vi "GUI_Bella_Control_Center_OFI.vi"() -> ()   [LabVIEW 2020]
uses:
  Shared/GUI_Template/GUI_master/tcp_new_data_event.ctl
  Shared/GUI_Template/GUI_master/tcp new data cluster.ctl
  GUI_TestStand/Fire button.ctl
  Device Drivers/DG645/subVIs/TriggerSource_TypDef.ctl
  <vilib>/Utility/config.llb/Write Key (I32).vi
  <vilib>/Platform/browser.llb/Open URL in Default Browser (string).vi
  <vilib>/Utility/config.llb/NI_LVConfig.lvlib
panel:
  in  "value5::42":dbl=0.006 caption="1BL-2BL-\nSplitter-Rpcnt" min=-9999999.0 max=9999999.0 format="%#_6p"
  in  "value6::43":bool=TRUE caption="GhostFoil-In"
  in  "value5::43":bool=TRUE caption="1BL-Energy\nMeter-In"
  in  "value4::43":bool=TRUE caption="2BLFoil-In"
  in  "value3::43":bool=TRUE caption="1BLFoil-In"
  in  "value2::43":bool=TRUE caption="ClunkerIn"
  out "CurrentStatus":string
  in  "MoveStage":bool
  in  "Position.Ch1::44":dbl caption="Current Position" min=0.0 max=150.0
  in  "GUIdevice 44":string="STAGE-LT-Megattenuator"
  in  "GUIdevice 43":string="MANPAR-BELLA-OFI-Boolean"
  in  "GUIdevice 42":string="MANPAR-BELLA-OFI"
  in  "Pressure.device 2::39":dbl caption="Dopant pressure\nLow1down" min=-20.0 max=500.0 format="%.3f"
  out "HPD2 to match HPD":dbl
  in  "Save screenshots":bool
  out "error out":errorcluster
  out "Hpd pos for jet exit":dbl
  in  "value2::42":dbl=276.0 caption="jet exit on hpd for hexX=0" min=-9999999.0 max=9999999.0
  in  "GUIdevice 41":string="STAGE-PL1-JetLength"
  in  "position::41":dbl caption="Jet Length pos" min=0.0 max=50.0 format="%.1f"
  out "lp mode HPDplane\n - HPD ref pos":dbl
  out "height above jet":dbl
  in  "value3::42":dbl=2.6 caption="zpos for 0 above jet" min=-9999999.0 max=9999999.0
  out "HPD - focus":dbl
  in  "value1::42":dbl=230.0 caption="focus on HPD" min=-9999999.0 max=9999999.0
  out "1BL delay (ns)\n+ is 1BL after 2BL":dbl
  in  "Position.Axis 1::8":dbl caption="1BL delay (mm)" min=-500.0 max=500.0 format="%.1f"
  in  "GUIdevice 8":string="STAGE-LT-1BLDelay"
  in  "value4::42":dbl=0.006 caption="JetOnTime" min=-9999999.0 max=9999999.0 format="%#_6p"
  in  "Position.Channel 5::25":dbl caption="SMFiber (45in, 1out)" min=-60.0 max=55.0 format="%.1f"
  in  "value1::43":bool=TRUE caption="GasJetOn"
  in  "value0::43":bool=TRUE caption="ShotControl"
  in  "Thales.DIAG_CU_Output_Percent_1::37":dbl caption="Amp2 att (%)" min=1.0 max=100.0 step=500.0 format="%.2f"
  in  "GUIdevice 37":string="SVE-LT-Thales"
  in  "Pressure.device 1::39":dbl caption="Hydrogen pressure\nHigh500" min=-20.0 max=500.0 format="%.3f"
  in  "GUIdevice 39":string="PRC-PL1-HighPressure"
  in  "Scan":T1(ring)
  in  "LogTable":bool
  in  "New Google\nExpLog for new day?":bool=TRUE
  out "standard output":string
  in  "Create Log":bool caption="LogTable"
  in  "GUIdevice 38":string="STAGE-2BL-Compressor"
  in  "Position.Axis 1::38":dbl caption="Comp2 Translation" min=0.0 max=20.0 format="%.3f"
  in  "Position.Channel 5::31":T2(ring) caption="FROG foil"
  in  "Position.Channel 2::31":T2(ring) caption="Little Rick"
  in  "AnalogOutput.Channel 1::36":dbl caption="M4A att (V)" min=0.0 max=5.0 step=500.0 format="%.2f"
  in  "GUIdevice 36":string="ATT-2BL-M4A"
  in  "GUIdevice 35":string="ATT-2BL-DM"
  in  "AnalogOutput.Channel 1::35":dbl caption="2BL DM att (V)" min=0.0 max=5.0 step=500.0 format="%.2f"
  in  "Step size 2":dbl=20.0 caption="Step size" min=-22.0 max=22.0
  in  "Position.Axis 4::33":dbl caption="Holy M V F4" min=-100000.0 max=100000.0 step=500.0
  in  "Position.Axis 3::33":dbl caption="Holy M H F3" min=-1000000.0 max=1000000.0 step=500.0
  in  "Position.Axis 2::33":dbl caption="Bessel M3 V F2" min=-100000.0 max=100000.0 step=500.0
  in  "Position.Axis 1::33":dbl caption="Bessel M3 H F1" min=-100000.0 max=100000.0 step=500.0
  in  "GUIdevice 33":string="MCD-PL1-picosOFI1"
  in  "Delay.Ch B::32":dbl caption="jet open time B" min=-0.1 max=0.1 format="%.3p"
  in  "Delay.Ch A::32":dbl caption="jet open A" min=-0.1 max=0.1 format="%.3p"
  in  "GUIdevice 32":string="DDG-AA-SRSGasJet-645"
  in  "position::6":dbl caption="LPmode stage long (605 safe)" min=0.0 max=605.0 format="%.1f"
  in  "GUIdevice 6":string="STAGE-PL1-LPmodeLong"
  in  "EnableMotor::6":bool caption="LPmode motor \nstatus"
  in  "GUIdevice 4":string="STAGE-PL1-Capstage1"
  in  "GUIdevice 31":string="1WIRE-BELLA-Flipper"
  in  "Amplitude.Ch GH::10":dbl=-1.631e-06 caption="Shot Shutter V" min=0.5 max=5.0 format="%.1f"
  in  "Rate (Hz)":dbl=0.3
  out "Crystal2":enum16{"In", "Out", "Unknown"}(ring)
  in  "wangle::28":dbl caption="w" min=-2.0 max=2.0 step=0.01 format="%.5f"
  in  "vangle::28":dbl caption="v" min=-5.0 max=5.0 step=0.01 format="%.5f"
  in  "uangle::28":dbl caption="u" min=-1.0 max=1.0 step=0.01 format="%.5f"
  in  "ypos::28":dbl caption="y" min=-3.0 max=3.0 step=0.01 format="%.5f"
  in  "zpos::28":dbl caption="z" min=-12.5 max=12.5 step=0.01 format="%.5f"
  in  "xpos::28":dbl caption="x" min=-0.5 max=0.5 step=0.01 format="%.5f"
  in  "GUIdevice 28":string="HEX-PL1-2"
  in  "Position.Channel 1::25":dbl caption="LPmode kicker (~1in, 75out)" min=-75.0 max=79.0 format="%.1f"
  in  "GUIdevice 25":string="STAGE-PL1-Smaract"
  in  "Heater Alignment Directions":bool
  in  "Position.Axis 3::15":dbl caption="XY" min=-3.0 max=16.0 format="%.4f"
  in  "Position.Axis 2::15":dbl caption="Y" min=-3.0 max=17.0 format="%.4f"
  in  "Position.Axis 1::15":dbl caption="X" min=-3.0 max=13.0 format="%.4f"
  in  "GUIdevice 24":string="STAGE-HEAT-TL1"
  in  "Encoder position::23":dbl caption="position HPD2" min=0.0 max=600.0 format="%.1f"
  in  "position::3":dbl caption="position HPD" min=0.0 max=600.0 format="%.1f"
  in  "GUIdevice 23":string="STAGE-HPD-Far"
  in  "GUIdevice 22":string="MANPAR-BELLA-FireCont"
  in  "Allow Fire Continues":bool
  out "Fire continues Indicator":bool caption="firing"
  in  "Fire Button":T3=TRUE
  in  "Trigger.Source::10":T4 caption="SRS Trigger Mode"
  out "Absolute discharge timing":dbl caption="delay from pk" format="%#.3p"
  in  "Delay.Ch E::17":dbl caption="Timing box" min=-0.1 max=0.1 format="%.3p"
  in  "value0::22":bool caption="Fire continuosly"
  in  "GUIdevice 15":string="MCD-HEAT-ESP1"
  in  "GUIdevice 17":string="DDG-AA-SRS0"
  out "error IO 2":errorcluster
  out "fire::10":string
  out "tcp data event":T5
  in  "UDP error message":string
  in  "GUIdevice 13":string="DDG-AA-SRS2"
  in  "GUIdevice 2":string="MANPAR-BELLA-General"
  in  "GUIdevice 10":string="DDG-AA-ShotCntrl"
  in  "GUIdevice 1":string="HEX-PL1-1"
  in  "GUIdevice 3":string="STAGE-HPD-Tel"
  in  "<command>::1":bool caption="ABORT\nHEXAPOD"
  in  "Step size":dbl min=-22.0 max=22.0 format="%.5f"
  in  "wangle::1":dbl caption="w (F11 F12)" min=-6.0 max=6.0 step=0.01 format="%.5f"
  in  "vangle::1":dbl caption="v (F9 F10)" min=-6.0 max=6.0 step=0.01 format="%.5f"
  in  "uangle::1":dbl caption="u (F7 F8)" min=-6.0 max=6.0 step=0.01 format="%.5f"
  in  "ypos::1":dbl caption="y (F3 F4)" min=-8.0 max=8.0 step=0.01 format="%.5f"
  in  "zpos::1":dbl caption="z (PgU PgD)" min=-12.0 max=15.0 step=0.01 format="%.5f"
  in  "xpos::1":dbl caption="x (F1 F2)" min=-25.0 max=22.0 step=0.01 format="%.5f"
  in  "Position.Axis 1::9":dbl caption="Comp1 Translation" min=-50.0 max=50.0 format="%.3f"
  in  "GUIdevice 9":string="STAGE-1BL-Compression"
  in  "stop":bool
  # "BELLA CONTROL CENTER"
  # "HEX 1 JET"
  # "HEX 2 Axicon"
  # "PICOS"
  # "DG"
  # "Jet"
  # "Discharge timing (s)"
  # "1wire"
  # "Heater timing (s)"
  # "\"-x\" is laser propagation direction"
  # "Scan"
  # "HPD Stage"
  # "PL1 stages"
  # "Megattenuator Stage"
  # "needs manpar-bella-ofi on\nMANPAR-BELLA-OFI-Boolean"
  # "Attenuate"
  # "OUT"
  # "IN"
  # "Compressors"
  # "Heater Alignment"
  # "Heat ESP0"
  # "Heat ESP1"
  # "Heat Pico"
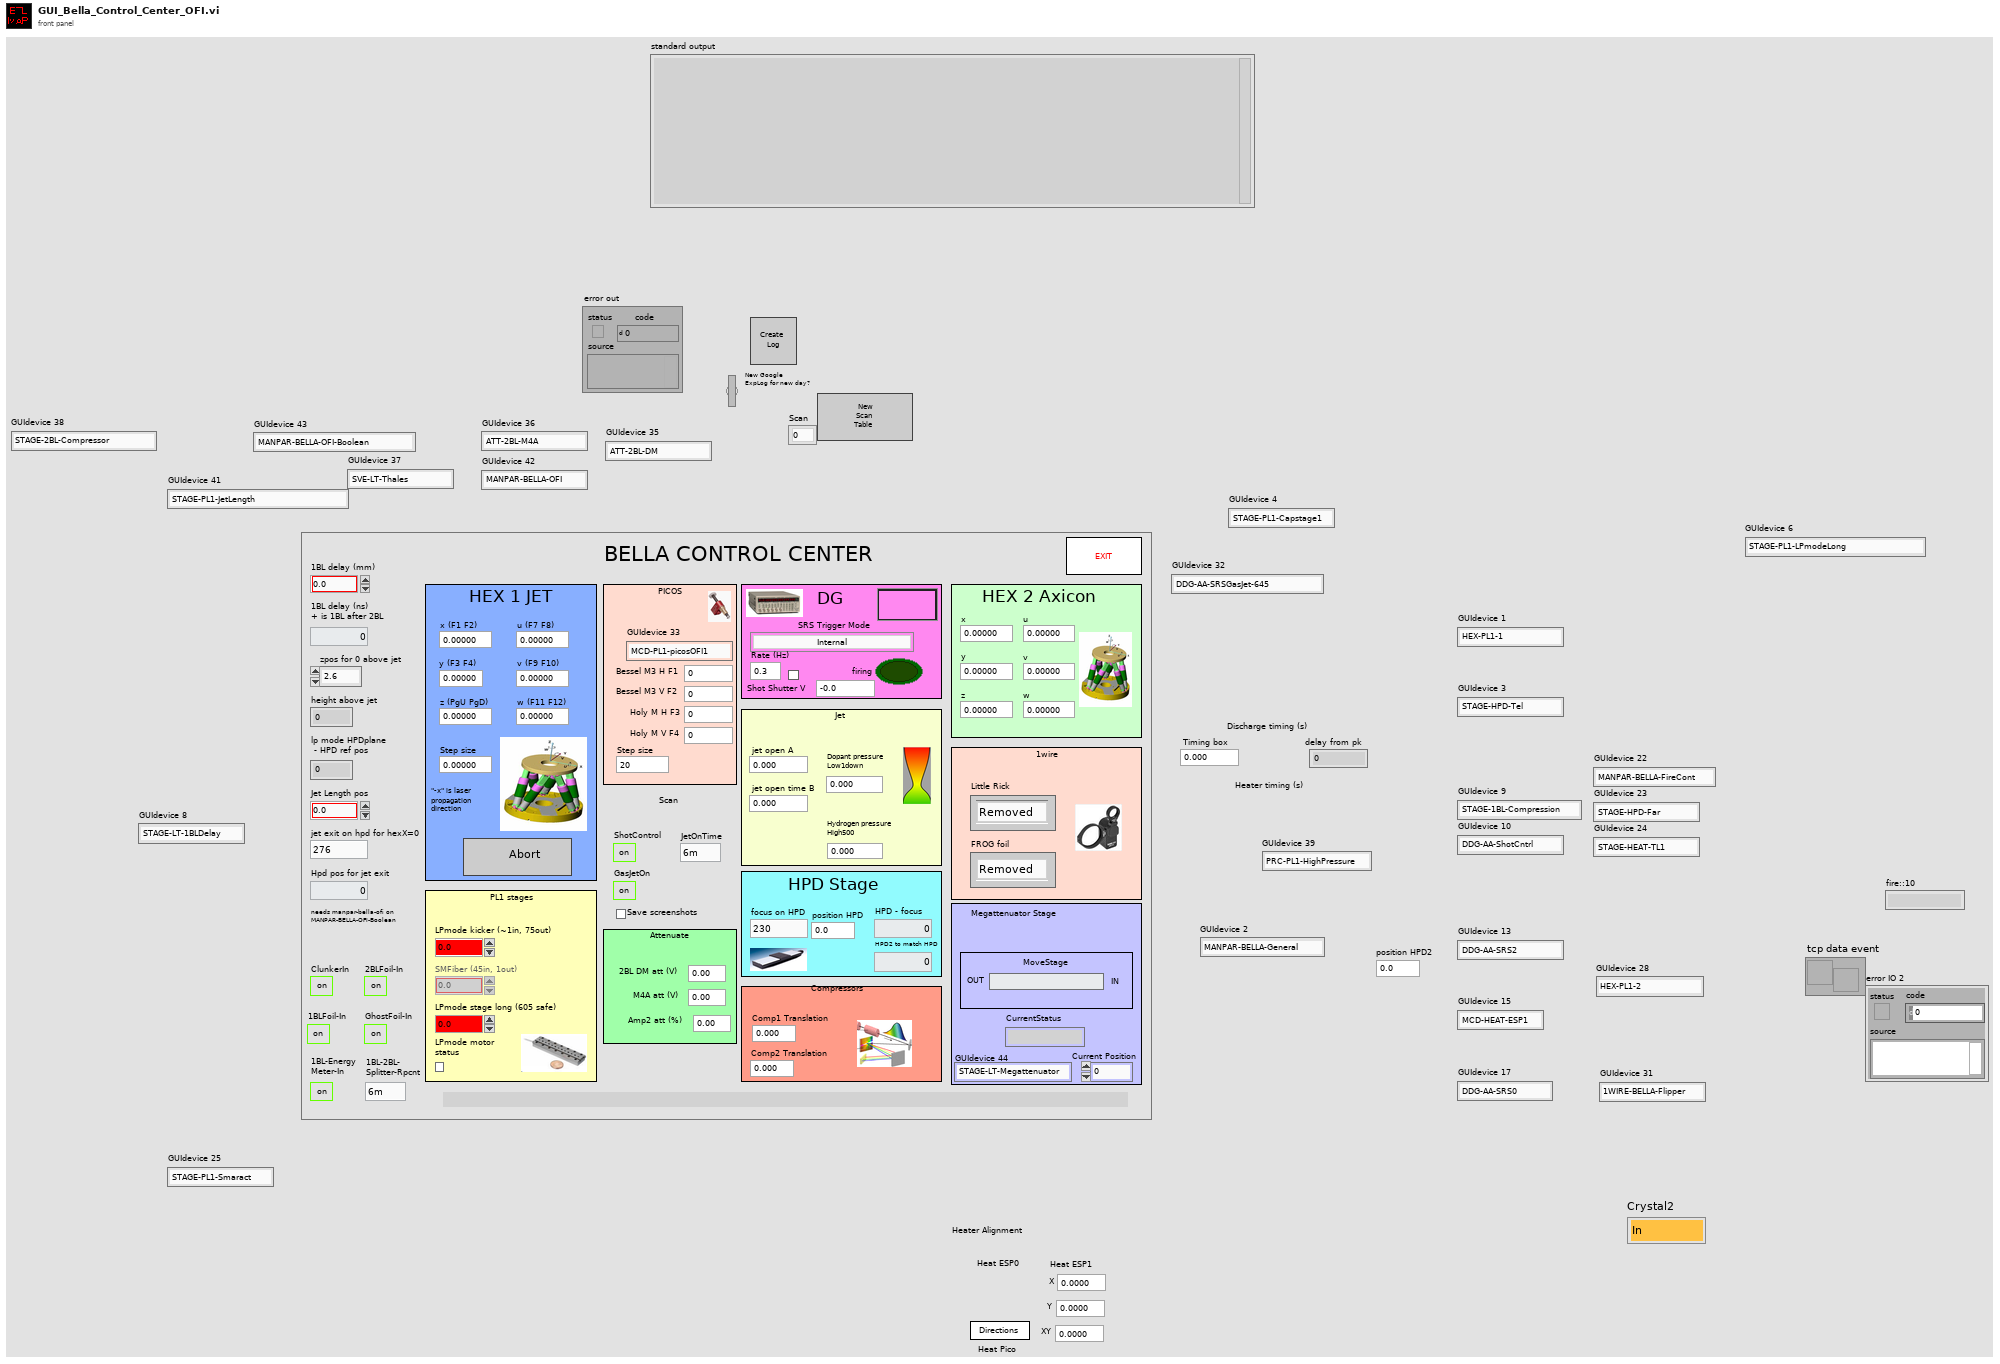
[diagram p1: front panel]
types:
  T1 = enum16{"0", "1", "2", "3", "4", "5", "6", "7", "8", "9", "10", "11", "12", "13", "14", "15", "16", "17", "18", "19", "20", "21", "22", "23", "24", "25", "26", "27", "28", "29", "30", "31", "32", "33", "34", "35", "36", "37", "38", "39", "40", "41", "42", "43", "44", "45", "46", "47", "48", "49", "50", "51", "52", "53", "54", "55", "56", "57", "58", "59", "60", "61", "62", "63", "64", "65", "66", "67", "68", "69", "70", "71", "72", "73", "74", "75", "76", "77", "78", "79", "81", "82", "83", "84", "85", "86", "87", "88", "89", "90", "91", "92", "93", "94", "95", "96", "97", "98", "99", ""}
  T2 = enum16{"Removed", "Inserted", "Unknown", "Moving"}
  T3 = typedef "Fire button.ctl" = bool
  T4 = typedef "TriggerSource_TypDef.ctl" = enum16{"Internal", "External rising edges", "External falling edges", "Single shot external rising edges", "Single shot external falling edges", "Single shot", "Line"}
  T5 = typedef "tcp_new_data_event.ctl" = refnum<user-event>
  T6 = typedef "tcp new data cluster.ctl" = cluster{"EventEnum":enum16{"new data", "connection status update"}, "Device name":string}
  T7 = enum8{"Enabled", "Disabled", "Disabled and Grayed Out"}
  T8 = enum32{"invalid app kind", "Development System", "Run Time System", "Student Edition", "Embedded LabVIEW", "Evaluation", "Custom"}
  T9 = enum32{"Invalid", "Standard", "Closed", "Hidden", "Minimized", "Maximized"}
  T10 = typedef "imagedata.ctl" = cluster{"image type":i32, "image depth":i32, "image":u8[], "mask":u8[], "colors":u32[], "Rectangle":cluster{"left":i16, "top":i16, "right":i16, "bottom":i16}}
  T11 = typedef "NI_LVConfig.lvlib/Config Data RefNum.ctl" = refnum<k1>
  T12 = cluster{"Core":cluster{"Current VI Reference":refnum<vi>, "Close Panel on Exit?":bool}, "Heater timing offset":dbl, "Discharge timing offset":dbl, "Jet trigger":bool, "Tik1":u32, "Tik2":u32, "Fire Continues Allowed":bool}
  T13 = cluster{"Current VI Reference":refnum<vi>, "Close Panel on Exit?":bool}
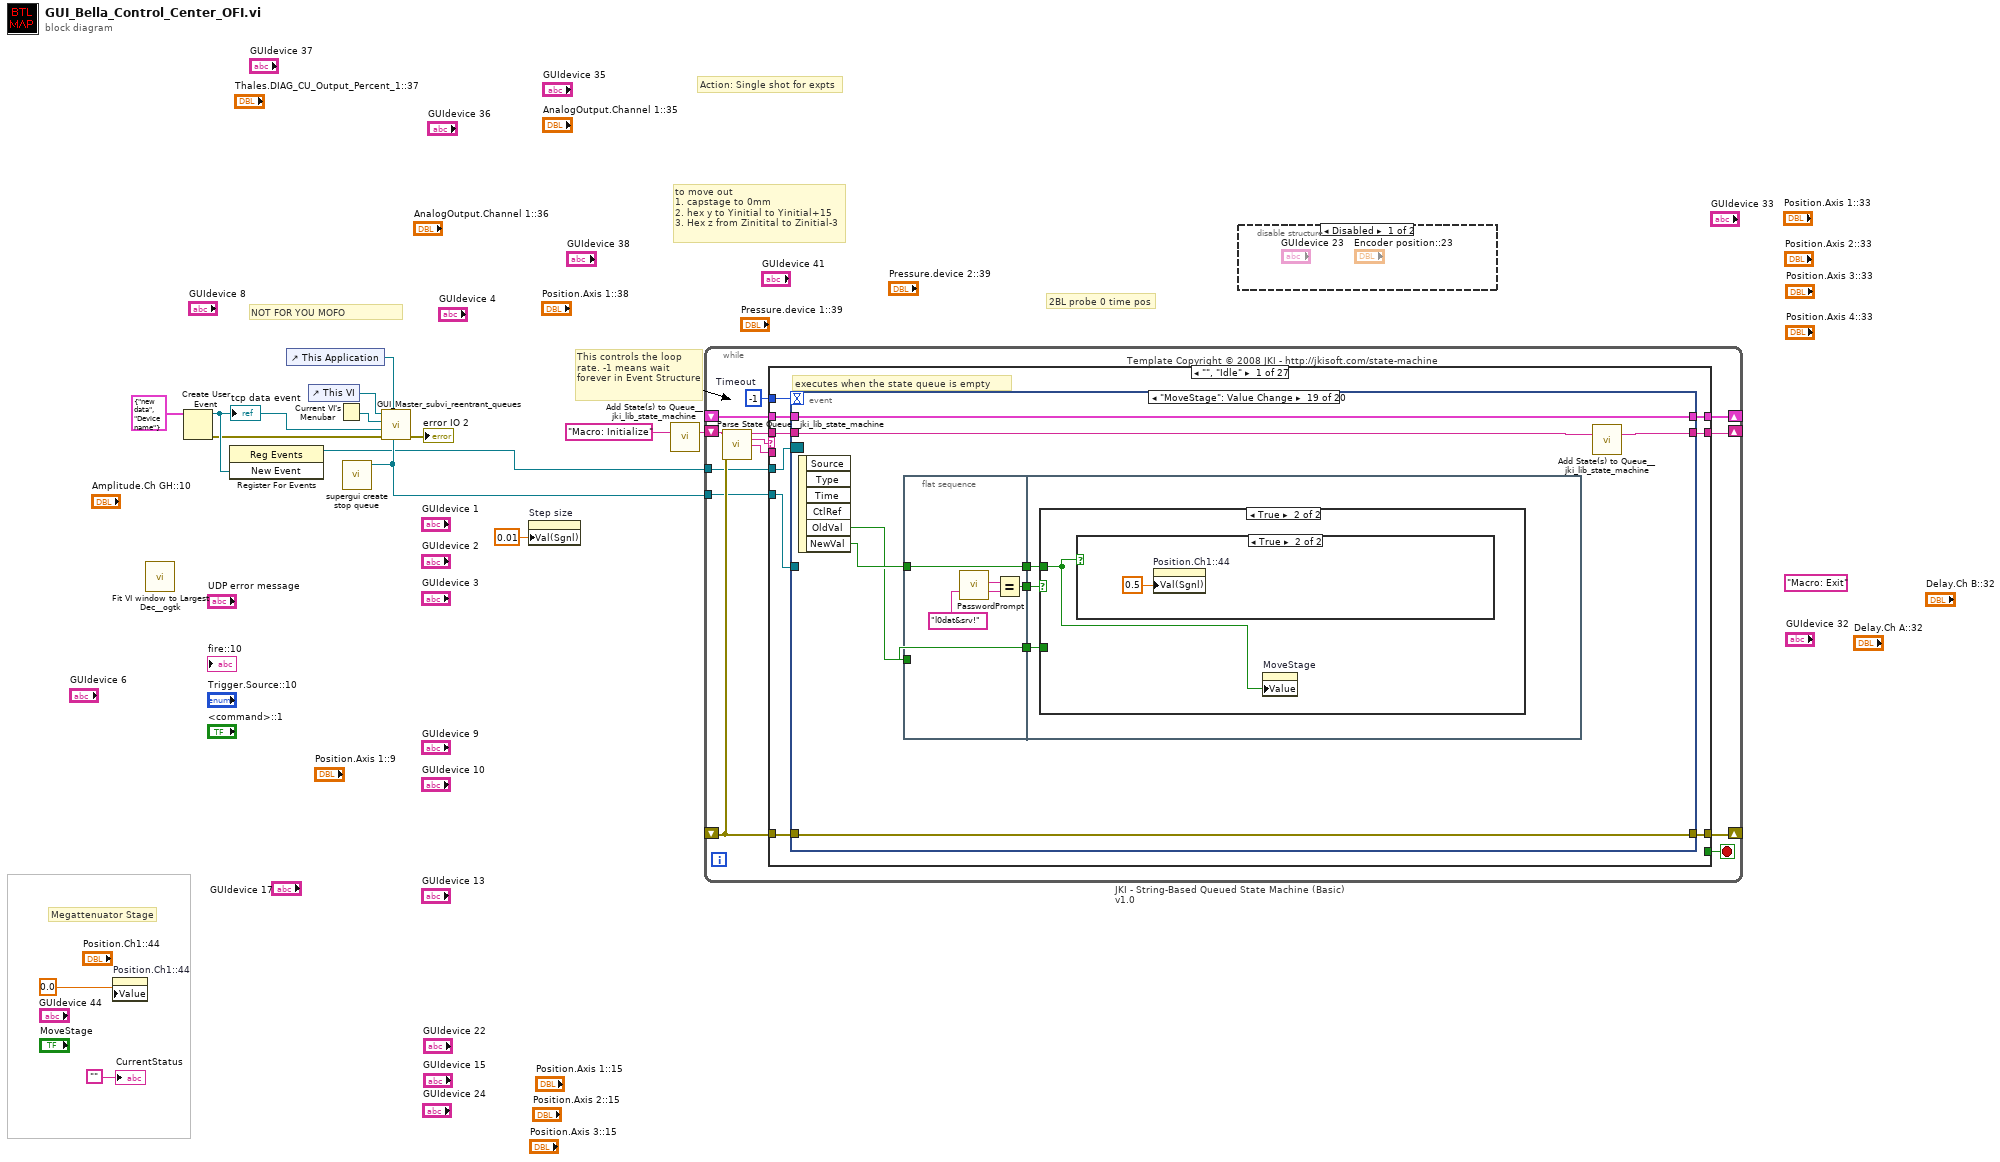
[diagram p0: block diagram]
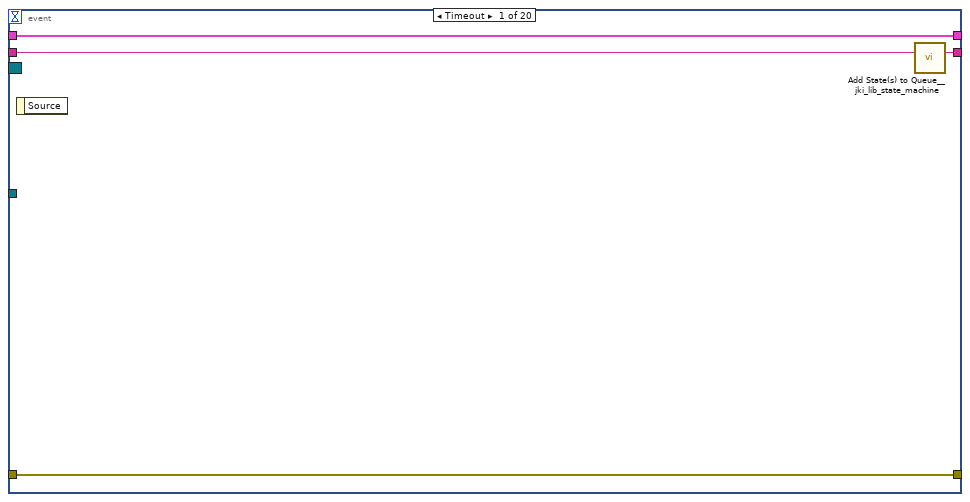
[diagram p3: hidden frame]
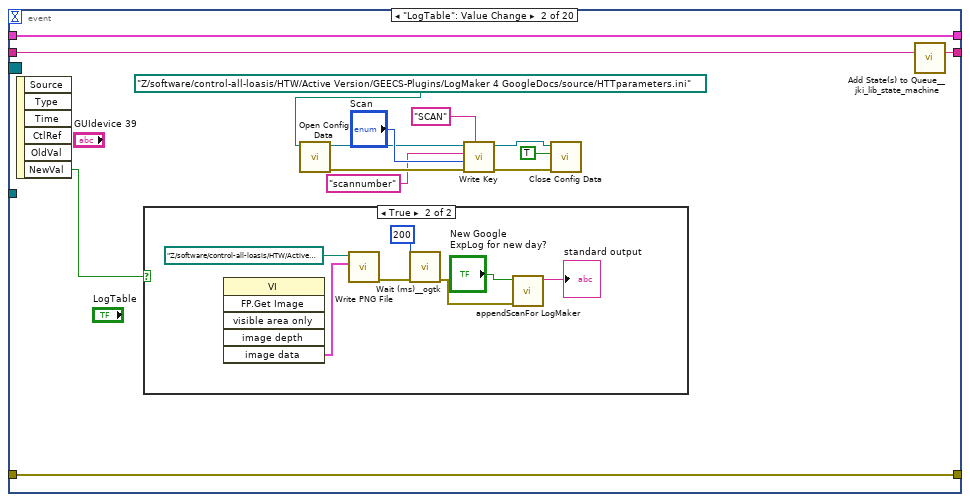
[diagram p4: hidden frame]
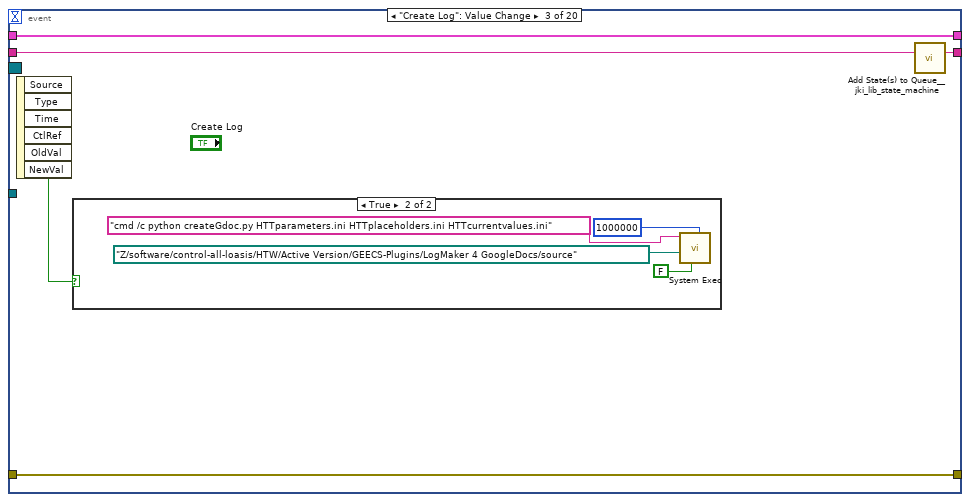
[diagram p6: hidden frame]
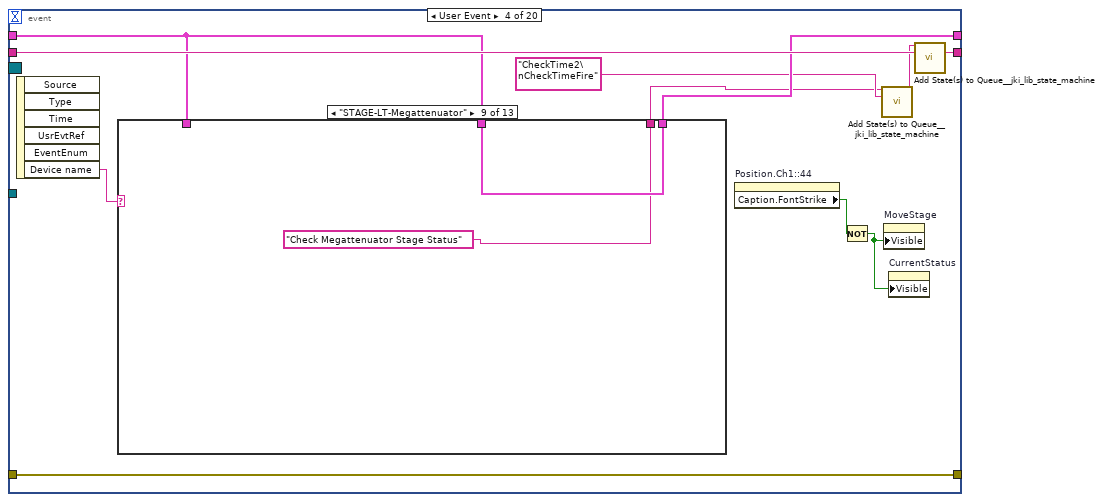
[diagram p8: hidden frame]
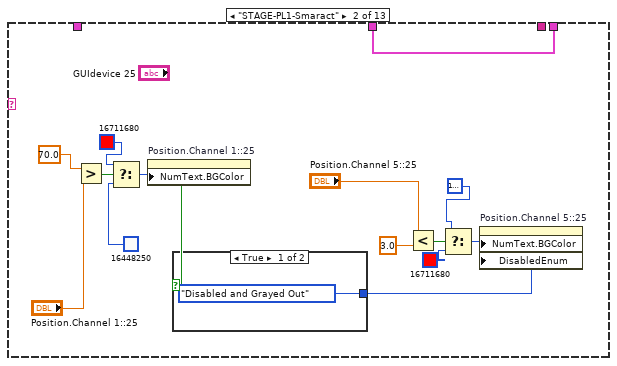
[diagram p10: hidden frame]
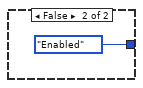
[diagram p11: hidden frame]
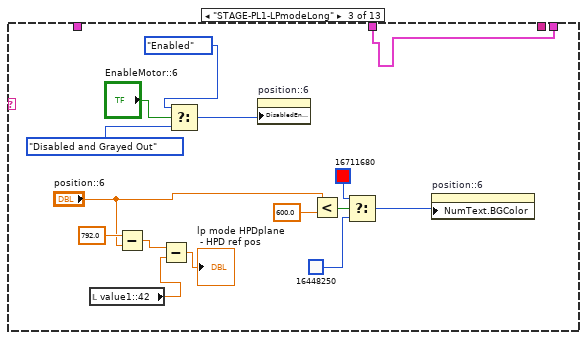
[diagram p12: hidden frame]
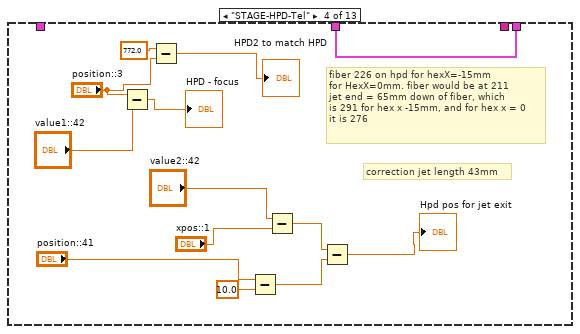
[diagram p13: hidden frame]
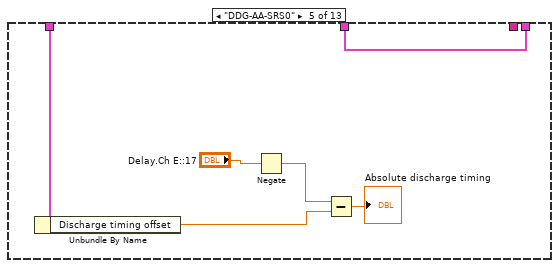
[diagram p14: hidden frame]
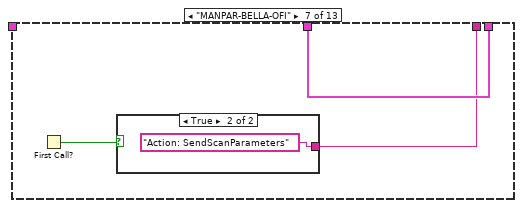
[diagram p16: hidden frame]
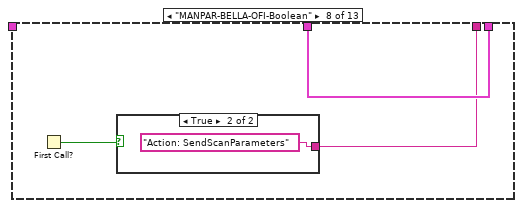
[diagram p18: hidden frame]
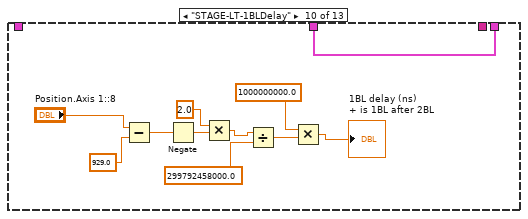
[diagram p20: hidden frame]
diagram:
  (unwired) "Macro: Exit"
  # "Megattenuator Stage"
  # "2BL probe 0 time pos"
  # "Action: Single shot for expts"
  # "to move out\n1. capstage to 0mm\n2. hex y to Yinitial to Yinitial+15\n3. Hex z from Zinitital to Zinitial-3"
  # "This controls the loop rate. -1 means wait forever in Event Structure"
  # "NOT FOR YOU MOFO"
  n1 = property on="Position.Ch1::44" class="DigNum (strict)"("Value"=0.0 ("Position.Ch1::44")) -> ()  [unwired: 2 in, 2 out]
  n2 = call <userlib>:"Fit VI window to Largest Dec__ogtk.vi"() -> ()  [unwired: 6 in, 2 out]
  n3 = Create User Event(user event datatype=T6 {"EventEnum"=enum."new data", "Device name"="Device name"} ("New Event")) -> (user event=w13:refnum<user-event>, error out=w12:errorcluster)  [unwired: 1 in]
  "tcp data event" <- w13
  n4 = register-events(w13) -> (reference out=w3:refnum<event-registration>)  [unwired: 2 in, 1 out]
  n5 = control-ref of="This Application"() -> (w14:refnum<vi>)
  n6 = control-ref of="This VI"() -> (w7:refnum<vi>)
  n7 = Current VI's Menubar() -> (w10:refnum<k9>)
  n8 = call "supergui create stop queue.vi"() -> ("STOP Queue out"=w4:refnum<queue>)  [unwired: 11 in]
  n9 = call "GUI_Master_subvi_reentrant_queues.vi"("STOP Queue in"=w4, "This Application"=w14, "error in (no error)"=w12, "tcp data event"=w13, "Caller menu reference"=w10, "Caller VI ref"=w7) -> ("error out"=→"error IO 2":errorcluster)  [unwired: 5 in]
  n10 = property on="Step size" class="DigNum (strict)"("Val(Sgnl)"=0.01 ("Value (Signaling)")) -> ()  [unwired: 2 in, 2 out]
  n11 = call <vilib>:"Add State(s) to Queue__jki_lib_state_machine.vi"("State(s) in (\"\")"="Macro: Initialize") -> ("States Out"=w5:string)  [unwired: 14 in]
  n12 = while "JKI - String-Based Queued State Machine (Basic) v1.0" {
    shift-right: [w20] -> _
    shift-left: _ -> [w19]
    shift-right: [w23] -> _
    shift-left: _ -> [w17]
    shift-right: [w22] -> _
    shift-left: w5 -> [w24]
    tunnel: w3 -> [w16]
    tunnel: w4 -> [w15]
    stop <- w21 stop-if-true
    w18 = -1  # Timeout
    # "Template Copyright © 2008 JKI - http://jkisoft.com/state-machine"
    n13 = call <vilib>:"Parse State Queue__jki_lib_state_machine.vi"("State Queue"=w24, "Error In (no error)"=w17) -> ("Remaining States"=w26:string, "Current State"=w27:string, "Arguments"=w25:string)  [unwired: 11 in]
    n14 = case shown="\"\", \"Idle\"" w27 {
      selector: w27 -> [_ _ w338 _ _ _ _ _ _ _ _ _ _ _ _ _ _ _ _ _ _ _ _ _ _ _ _]
      tunnel: w26 -> [w36 w337 w342 w360 w366 w371 w375 w386 w392 w396 w400 w406 w417 w443 w448 w461 w465 w471 w480 w517 w528 w540 w552 w561 w565 w574 w580]
      tunnel: w25 -> [_ _ _ _ _ _ _ _ _ _ _ w401 w411 _ _ _ _ _ _ _ _ _ _ _ _ _ _]
      tunnel: w19 -> [w34 w334 w340 w351 w363 w369 w372 _ w387 w393 w398 w404 w413 w440 w445 w458 w462 w468 w477 w505 w524 w534 w549 w559 w562 w571 w577]
      tunnel: [w33 w335 w344 w357 errorcluster {"status"=FALSE, "code"=0, "source"=""} ("error out") w368 w373 w383 w388 w394 w397 w402 w414 w441 w446 w459 w463 w469 w478 w515 w522 w529 w550 w556 w563 w572 w578] -> w23
      tunnel: w17 -> [w32 w335 w343 w357 w362 w368 w373 w383 w389 w394 w397 w403 w415 w441 w446 w459 w463 w469 w478 w515 w526 w530 w550 w557 w563 w572 w578]
      tunnel: [w35 w336 w341 w359 w365 w370 w374 w385 w391 w395 w399 w405 w416 w442 w447 w460 w464 w470 w479 w516 w527 w539 w551 w560 w564 w573 w579] -> w22
      tunnel: [_ _ _ _ _ TRUE _ _ _ _ _ _ _ _ _ _ _ _ _ _ _ _ _ _ _ _ _] -> w21
      tunnel: [w28 w334 w340 w358 w363 w369 w372 w384 w387 w393 w398 w404 w413 w440 w445 w458 w462 w468 w477 w514 w524 w533 w548 w559 w562 w571 w577] -> w20
      tunnel: w18 -> [w31 _ _ _ _ _ _ _ _ _ _ _ _ _ _ _ _ _ _ _ _ _ _ _ _ _ _]
      tunnel: w16 -> [w30 _ _ _ _ _ _ _ _ _ _ _ _ _ _ _ _ _ _ _ _ _ _ _ _ _ _]
      tunnel: w15 -> [w29 _ _ _ _ _ _ _ _ _ _ _ _ _ _ w450 _ _ _ _ _ _ _ _ _ _ _]
      frame "", "Idle" {
        # "executes when the state queue is empty"
        n15 = event shown="[18] \"MoveStage\": Value Change" {
          selector: w30 -> [_ _ _ _ _ _ _ _ _ _ _ _ _ _ _ _ _ _ _ _]
          dyn-events: _ -> [_ _ _ _ _ _ _ _ _ _ _ _ _ _ _ _ _ _ _ _]
          timeout: w31 -> [_ _ _ _ _ _ _ _ _ _ _ _ _ _ _ _ _ _ _ _]
          tunnel: w36 -> [w40 w54 w66 w81 w182 w184 w189 w199 w209 w219 w229 w239 w248 w256 w265 w288 w298 w305 w307 w333]
          tunnel: [w39 w53 w65 w80 w181 w185 w190 w200 w210 w220 w230 w240 w249 w256 w264 w288 w298 w305 w306 w332] -> w35
          tunnel: w34 -> [w37 w51 w63 w77 w179 w187 w192 w202 w212 w222 w232 w242 w251 w255 w267 w289 w299 w304 w314 w330]
          tunnel: [w38 w52 w64 w79 w180 w186 w191 w201 w211 w221 w231 w241 w250 w253 w270 w287 w297 w303 w313 w331] -> w33
          tunnel: w32 -> [w38 w52 w64 w79 w180 w186 w191 w201 w211 w221 w231 w241 w250 w254 w269 w287 w297 w303 w313 w331]
          tunnel: [w37 w51 w63 w76 w179 w187 w192 w202 w212 w222 w232 w242 w251 w255 w268 w289 w299 w304 w314 w330] -> w28
          tunnel: w29 -> [_ _ _ _ _ _ _ _ _ _ _ _ _ _ _ _ _ _ _ _]
          event Timeout {
            n16 = event-data() -> ()  [unwired: 1 in, 1 out]
            n17 = call <vilib>:"Add State(s) to Queue__jki_lib_state_machine.vi"("State(s) in (\"\")"=w40) -> ("States Out"=w39:string)  [unwired: 14 in]
          }
          event "LogTable": Value Change {
            n18 = event-data() -> ("NewVal"=w41:bool)  [unwired: 1 in, 5 out]
            n19 = case shown="True" w41 {
              frame False {
              }
              frame True {
                n20 = invoke class="VI" method="FP.Get Image"() -> ("image data"=w61:T10)  [unwired: 6 in, 5 out]
                n21 = call <vilib>:"Write PNG File.vi"("image data"=w61, "path to PNG file"=path "Z:/software/control-all-loasis/HTW/Active Version/GEECS-Plugins/LogMaker 4 GoogleDocs/source/frontpanel.png" ("report file path")) -> ("error out"=w56:errorcluster)  [unwired: 8 in, 1 out]
                n22 = call <userlib>:"Wait (ms)__ogtk.vi"("error in (no error)"=w56, "milliseconds to wait"=u32 200 ("millisecond timer value")) -> ("error out"=w55:errorcluster)  [unwired: 8 in, 1 out]
                n23 = call "appendScanFor LogMaker.vi"("error in (no error)"=w55, "New Google\nExpLog for new day?"="New Google\nExpLog for new day?") -> ("standard output"=→"standard output":string)  [unwired: 9 in]
              }
            }
            n24 = call <vilib>:"Open Config Data.vi"("configuration file path"=path "Z:/software/control-all-loasis/HTW/Active Version/GEECS-Plugins/LogMaker 4 GoogleDocs/source/HTTparameters.ini") -> ("error out"=w48:errorcluster, "refnum"=w46:T11)  [unwired: 8 in, 1 out]
            n25 = call-poly <vilib>:"Write Key.vi"("section"="SCAN", "error in (no error)"=w48, "value"="Scan", "key"="scannumber", "refnum"=w46) -> ("error out"=w49:errorcluster, "refnum out"=w47:T11)  [unwired: 4 in, 1 out]
            n26 = call <vilib>:"Close Config Data.vi"("error in (no error)"=w49, "write file if changed (T)"=TRUE, "refnum"=w47) -> ()  [unwired: 7 in, 2 out]
            n27 = call <vilib>:"Add State(s) to Queue__jki_lib_state_machine.vi"("State(s) in (\"\")"=w54) -> ("States Out"=w53:string)  [unwired: 14 in]
          }
          event "Create Log": Value Change {
            n28 = event-data() -> ("NewVal"=w62:bool)  [unwired: 1 in, 5 out]
            n29 = case shown="True" w62 {
              frame False {
              }
              frame True {
                n30 = call <vilib>:"System Exec.vi"("expected output size  (4096)"=u32 1000000, "run minimized? (F)"=FALSE, "working directory"=path "Z:/software/control-all-loasis/HTW/Active Version/GEECS-Plugins/LogMaker 4 GoogleDocs/source", "command line"="cmd /c python createGdoc.py HTTparameters.ini HTTplaceholders.ini HTTcurrentvalues.ini") -> ()  [unwired: 4 in, 4 out]
              }
            }
            n31 = call <vilib>:"Add State(s) to Queue__jki_lib_state_machine.vi"("State(s) in (\"\")"=w66) -> ("States Out"=w65:string)  [unwired: 14 in]
          }
          event User Event {
            n32 = event-data() -> ("Device name"=w78:string)  [unwired: 1 in, 5 out]
            n33 = case shown="\"STAGE-LT-Megattenuator\"" w78 {
              tunnel: w77 -> [_ _ _ _ w129 _ _ _ _ _ _ _ _]
              tunnel: w77 -> [w82 w96 w113 w126 w127 w133 w136 w140 w143 w148 w155 w157 w177]
              tunnel: [w82 w96 w113 w126 w127 w133 w136 w140 w143 w148 w155 w157 w177] -> w76
              tunnel: [_ _ _ _ _ _ w135 w139 "Check Megattenuator Stage Status" ("State(s) in Front (\"\")") _ _ _ _] -> w73
              frame "False", Default {
              }
              frame "STAGE-PL1-Smaract" {
                n34 = Greater?(x=70.0 ("y"), y="Position.Channel 1::25") -> (0:w83:bool)
                n35 = Select(t=u32 16711680, s=w83, f=u32 16448250) -> (s? t:f=w93:u32)
                n36 = property on="Position.Channel 1::25" class="DigNum (strict)"("NumText.BGColor"=w93) -> ()  [unwired: 2 in, 2 out]
                n37 = case shown="True" w83 {
                  tunnel: [T7."Disabled and Grayed Out" ("Disabled") T7."Enabled" ("Disabled")] -> w84
                  frame True {
                  }
                  frame False {
                  }
                }
                n38 = Less?(x="Position.Channel 5::25", y=3.0) -> (x < y?=w89:bool)
                n39 = Select(t=u32 16777225, s=w89, f=u32 16711680) -> (s? t:f=w92:u32)
                n40 = property on="Position.Channel 5::25" class="DigNum (strict)"("NumText.BGColor"=w92, "DisabledEnum"=w84) -> ()  [unwired: 2 in, 2 out]
              }
              frame "STAGE-PL1-LPmodeLong" {
                n41 = local read "value1::42"() -> (w100:dbl)
                n42 = Subtract(x=792.0, y="position::6") -> (x-y=w101:dbl)
                n43 = Subtract(x=w101, y=w100) -> (x-y=→"lp mode HPDplane\n - HPD ref pos":dbl)
                n44 = Select(t=T7."Enabled" ("Disabled"), s="EnableMotor::6", f=T7."Disabled and Grayed Out" ("Disabled")) -> (s? t:f=w104:T7)
                n45 = property on="position::6" class="DigNum (strict)"("DisabledEnum"=w104) -> ()  [unwired: 2 in, 2 out]
                n46 = Less?(x="position::6", y=600.0) -> (x < y?=w112:bool)
                n47 = Select(t=u32 16711680, s=w112, f=u32 16448250) -> (s? t:f=w108:u32)
                n48 = property on="position::6" class="DigNum (strict)"("NumText.BGColor"=w108) -> ()  [unwired: 2 in, 2 out]
              }
              frame "STAGE-HPD-Tel" {
                # "correction jet length 43mm"
                # "fiber 226 on hpd for hexX=-15mm\nfor HexX=0mm. fiber would be at 211\njet end = 65mm down of fiber, which\nis 291 for hex x -15mm, and for hex x = 0\nit is 276"
                n49 = Subtract(x="position::3", y="value1::42") -> (x-y=→"HPD - focus":dbl)
                n50 = Subtract(x=772.0 ("y"), y="position::3") -> (x-y=→"HPD2 to match HPD":dbl)
                n51 = Subtract(x="position::41", y=10.0) -> (x-y=w118:dbl)
                n52 = Subtract(x="value2::42", y="xpos::1") -> (x-y=w119:dbl)
                n53 = Subtract(x=w119, y=w118) -> (x-y=→"Hpd pos for jet exit":dbl)
              }
              frame "DDG-AA-SRS0" {
                n54 = Unbundle By Name(w129) -> ("Discharge timing offset"=w128:dbl)
                n55 = Negate(x="Delay.Ch E::17") -> (-x=w130:dbl)
                n56 = Subtract(x=w130, y=w128) -> (x-y=→"Absolute discharge timing":dbl)
              }
              frame "STAGE-2BL-ProbeDelay" {
              }
              frame "MANPAR-BELLA-OFI" {
                n57 = First Call?() -> (First Call?: T/F=w134:bool)
                n58 = case shown="True" w134 {
                  tunnel: [_ "Action: SendScanParameters" ("State(s) in Front (\"\")")] -> w135
                  frame False {
                  }
                  frame True {
                  }
                }
              }
              frame "MANPAR-BELLA-OFI-Boolean" {
                n59 = First Call?() -> (First Call?: T/F=w138:bool)
                n60 = case shown="True" w138 {
                  tunnel: [_ "Action: SendScanParameters" ("State(s) in Front (\"\")")] -> w139
                  frame False {
                  }
                  frame True {
                  }
                }
              }
              frame "STAGE-LT-Megattenuator" {
              }
              frame "STAGE-LT-1BLDelay" {
                n61 = Subtract(x="Position.Axis 1::8", y=929.0) -> (x-y=w153:dbl)
                n62 = Negate(x=w153) -> (-x=w152:dbl)
                n63 = Multiply(x=2.0, y=w152) -> (x*y=w150:dbl)
                n64 = Divide(x=w150, y=299792458000.0) -> (x/y=w147:dbl)
                n65 = Multiply(x=1000000000.0, y=w147) -> (x*y=→"1BL delay (ns)\n+ is 1BL after 2BL":dbl)
              }
              frame "1WIRE-BELLA-Flipper" {
              }
              frame "HEX-PL1-2" {
                n66 = disable-structure shown="Disabled" {
                  disable-tunnel: "ypos::28" -> [w161 _]
                  frame Disabled {
                    n67 = Equal?(x=w161, y=15.6) -> (x = y?=w159:bool)
                    n68 = Equal?(x=-20.0 ("y"), y=w161) -> (x = y?=w163:bool)
                    n69 = case shown="False" w163 {
                      tunnel: [w167 enum16{"In", "Out"}."Out" ("sdfsdfs 2")] -> w158
                      tunnel: [w165 u32 16185078] -> w162
                      tunnel: w159 -> [w166 _]
                      frame False {
                        n70 = case shown="False" w166 {
                          tunnel: [enum16{"In", "Out", "Unknown"}."Unknown" ("sdfsdfs 2") enum16{"In", "Out"}."In" ("sdfsdfs 2")] -> w167
                          tunnel: [u32 16761154 ("Color Box") u32 16711680] -> w165
                          frame False {
                          }
                          frame True {
                          }
                        }
                      }
                      frame True {
                      }
                    }
                    "Crystal2" <- w158
                    n71 = property on="Crystal2" class="Enum (strict)"("RingText.FG Color"=w162, "RingText.BGColor"=w162) -> ()  [unwired: 2 in, 2 out]
                  }
                  frame Enabled {
                  }
                }
              }
              frame "HEX-PL1-1" {
                n72 = Subtract(x="value3::42", y="zpos::1") -> (x-y=→"height above jet":dbl)
              }
            }
            n73 = property on="Position.Ch1::44" class="DigNum (strict)"() -> ("Caption.FontStrike"=w72:bool)  [unwired: 2 in, 2 out]
            n74 = Not(x=w72) -> (.not. x?=w71:bool)
            n75 = call <vilib>:"Add State(s) to Queue__jki_lib_state_machine.vi"("State(s) in Front (\"\")"=w73, "State(s) in (\"\")"="CheckTime2\nCheckTimeFire" ("State(s) in Front (\"\")")) -> ("States Out"=w74:string)  [unwired: 13 in]
            n76 = property on="MoveStage" class="Bool (strict)"("Visible"=w71) -> ()  [unwired: 2 in, 2 out]
            n77 = property on="CurrentStatus" class="Str"("Visible"=w71) -> ()  [unwired: 2 in, 2 out]
            n78 = call <vilib>:"Add State(s) to Queue__jki_lib_state_machine.vi"("State(s) in Front (\"\")"=w74, "State(s) in (\"\")"=w81) -> ("States Out"=w80:string)  [unwired: 13 in]
          }
          event "stop": Value Change {
            # "Exit Button Value Change (pressed) Event\n(this executes Macro: Exit to terminate the VI)"
            n79 = event-data() -> ()  [unwired: 1 in, 6 out]
            n80 = call <vilib>:"Add State(s) to Queue__jki_lib_state_machine.vi"("State(s) in Front (\"\")"="Macro: Exit", "State(s) in (\"\")"=w182) -> ("States Out"=w181:string)  [unwired: 13 in]
          }
          event Value Change {
            n81 = event-data() -> ()  [unwired: 1 in, 6 out]
            n82 = call <vilib>:"Add State(s) to Queue__jki_lib_state_machine.vi"("State(s) in Front (\"\")"="Action: Fire" ("State(s) in Front (\"\")"), "State(s) in (\"\")"=w184) -> ("States Out"=w185:string)  [unwired: 13 in]
          }
          event "value0::43", "value1::43", "value4::42": Value Change {
            n83 = event-data() -> ()  [unwired: 1 in, 6 out]
            n84 = call <vilib>:"Add State(s) to Queue__jki_lib_state_machine.vi"("State(s) in Front (\"\")"="Action: SendScanParameters" ("State(s) in Front (\"\")"), "State(s) in (\"\")"=w189) -> ("States Out"=w190:string)  [unwired: 13 in]
          }
          event "value2::43": Value Change {
            n85 = event-data() -> ()  [unwired: 1 in, 6 out]
            n86 = local read "GUIdevice 43"() -> (w193:string)
            n87 = Select(t="on", s="value2::43", f="off") -> (s? t:f=w198:string)
            n88 = call "DefaultValue_Variable_MC.vi"("Variable In"="value2", "Default Value"=w198, "Device In"=w193) -> ()  [unwired: 1 in]
            n89 = call <vilib>:"Add State(s) to Queue__jki_lib_state_machine.vi"("State(s) in (\"\")"=w199) -> ("States Out"=w200:string)  [unwired: 14 in]
          }
          event "value3::43": Value Change {
            n90 = event-data() -> ()  [unwired: 1 in, 6 out]
            n91 = local read "GUIdevice 43"() -> (w204:string)
            n92 = Select(t="on", s="value3::43", f="off") -> (s? t:f=w208:string)
            n93 = call "DefaultValue_Variable_MC.vi"("Variable In"="value3", "Default Value"=w208, "Device In"=w204) -> ()  [unwired: 1 in]
            n94 = call <vilib>:"Add State(s) to Queue__jki_lib_state_machine.vi"("State(s) in (\"\")"=w209) -> ("States Out"=w210:string)  [unwired: 14 in]
          }
          event "value4::43": Value Change {
            n95 = event-data() -> ()  [unwired: 1 in, 6 out]
            n96 = local read "GUIdevice 43"() -> (w214:string)
            n97 = Select(t="on", s="value4::43", f="off") -> (s? t:f=w218:string)
            n98 = call "DefaultValue_Variable_MC.vi"("Variable In"="value4", "Default Value"=w218, "Device In"=w214) -> ()  [unwired: 1 in]
            n99 = call <vilib>:"Add State(s) to Queue__jki_lib_state_machine.vi"("State(s) in (\"\")"=w219) -> ("States Out"=w220:string)  [unwired: 14 in]
          }
          event "value5::43": Value Change {
            n100 = event-data() -> ()  [unwired: 1 in, 6 out]
            n101 = local read "GUIdevice 43"() -> (w224:string)
            n102 = Select(t="on", s="value5::43", f="off") -> (s? t:f=w228:string)
            n103 = call "DefaultValue_Variable_MC.vi"("Variable In"="value5", "Default Value"=w228, "Device In"=w224) -> ()  [unwired: 1 in]
            n104 = call <vilib>:"Add State(s) to Queue__jki_lib_state_machine.vi"("State(s) in (\"\")"=w229) -> ("States Out"=w230:string)  [unwired: 14 in]
          }
          event "value6::43": Value Change {
            n105 = event-data() -> ()  [unwired: 1 in, 6 out]
            n106 = local read "GUIdevice 43"() -> (w234:string)
            n107 = Select(t="on", s="value6::43", f="off") -> (s? t:f=w238:string)
            n108 = call "DefaultValue_Variable_MC.vi"("Variable In"="value6", "Default Value"=w238, "Device In"=w234) -> ()  [unwired: 1 in]
            n109 = call <vilib>:"Add State(s) to Queue__jki_lib_state_machine.vi"("State(s) in (\"\")"=w239) -> ("States Out"=w240:string)  [unwired: 14 in]
          }
          event "value5::42": Value Change {
            n110 = event-data() -> ()  [unwired: 1 in, 6 out]
            n111 = Number To Fractional String(number="value5::42", precision (6)=i16 4) -> (F-format string=w244:string)  [unwired: 2 in]
            n112 = call "DefaultValue_Variable_MC.vi"("Variable In"="value5", "Default Value"=w244, "Device In"="GUIdevice 42") -> ()  [unwired: 1 in]
            n113 = call <vilib>:"Add State(s) to Queue__jki_lib_state_machine.vi"("State(s) in (\"\")"=w248) -> ("States Out"=w249:string)  [unwired: 14 in]
          }
          event "Heater Alignment Directions": Value Change {
            n114 = event-data() -> ()  [unwired: 1 in, 6 out]
            n115 = case shown="True" "Heater Alignment Directions" {
              tunnel: w254 -> [w257 w260]
              tunnel: [w257 w259] -> w253
              frame False {
              }
              frame True {
                n116 = call-poly <vilib>:"Open URL in Default Browser.vi"("error in (no error)"=w260, "URL"="https://docs.google.com/document/d/1RMZp6W8Kkog2nkTymSjyZ2bh9D7Vo4bxhvGgn3Ut4KE/edit") -> ("error out"=w259:errorcluster)  [unwired: 4 in, 1 out]
              }
            }
          }
          event "Allow Fire Continues": Value Change {
            n117 = event-data() -> ()  [unwired: 1 in, 6 out]
            n118 = Unbundle By Name(w267) -> ("Fire Continues Allowed"=w266:bool)
            n119 = case shown="True" "Allow Fire Continues" {
              tunnel: [w271 w278] -> w270
              tunnel: "Allow Fire Continues" -> [_ w277]
              tunnel: w269 -> [w271 w276]
              tunnel: w266 -> [w272 w275]
              tunnel: [w272 w273] -> w262
              tunnel: [_ "Initilize Fire Continues" ("State(s) in Front (\"\")")] -> w261
              frame False {
              }
              frame True {
                n120 = case shown="False" w275 {
                  tunnel: [w284 w285] -> w278
                  tunnel: w277 -> [w283 _]
                  tunnel: w276 -> [w282 w285]
                  tunnel: [w279 FALSE] -> w273
                  frame False {
                    n121 = call "Password"("Enable"=w283, "error in (no error)"=w282) -> ("Password"=w281:string, "error out"=w284:errorcluster)  [unwired: 15 in, 1 out]
                    n122 = Equal?(x=w281, y="fire") -> (x = y?=w279:bool)
                  }
                  frame True {
                  }
                }
              }
            }
            n123 = Bundle By Name(cluster=w267, "Fire Continues Allowed"=w262) -> (w268:T12)
            n124 = call <vilib>:"Add State(s) to Queue__jki_lib_state_machine.vi"("State(s) in Front (\"\")"=w261, "State(s) in (\"\")"=w265) -> ("States Out"=w264:string)  [unwired: 13 in]
          }
          event "Step size": Value Change {
            n125 = event-data() -> ("NewVal"=w290:dbl)  [unwired: 1 in, 5 out]
            n126 = property on="uangle::1" class="DigNum (strict)"("Increment"=w290) -> ()  [unwired: 2 in, 2 out]
            n127 = property on="vangle::1" class="DigNum (strict)"("Increment"=w290) -> ()  [unwired: 2 in, 2 out]
            n128 = property on="xpos::1" class="DigNum (strict)"("Increment"=w290) -> ()  [unwired: 2 in, 2 out]
            n129 = property on="zpos::1" class="DigNum (strict)"("Increment"=w290) -> ()  [unwired: 2 in, 2 out]
            n130 = property on="wangle::1" class="DigNum (strict)"("Increment"=w290) -> ()  [unwired: 2 in, 2 out]
            n131 = property on="ypos::1" class="DigNum (strict)"("Increment"=w290) -> ()  [unwired: 2 in, 2 out]
          }
          event "Step size 2": Value Change {
            n132 = event-data() -> ("NewVal"=w291:dbl)  [unwired: 1 in, 5 out]
            n133 = control-ref of="Position.Axis 1::33"() -> (w296:refnum<vi>)
            n134 = control-ref of="Position.Axis 2::33"() -> (w295:refnum<vi>)
            n135 = control-ref of="Position.Axis 4::33"() -> (w293:refnum<vi>)
            n136 = control-ref of="Position.Axis 3::33"() -> (w294:refnum<vi>)
            n137 = Build Array(w296, w295, w294, w293) -> (w292:refnum<vi>[])
            n138 = for {
              tunnel: w292 -> [w301] mode=indexing
              tunnel: w291 -> [w300]
              n139 = property on="Property Node" class="DigNum (strict)"(reference=w301, "Increment"=w300) -> ()  [unwired: 1 in, 2 out]
            }
          }
          event Value Change {
            n140 = event-data() -> ()  [unwired: 1 in, 6 out]
            n141 = property on="value0::22" class="Bool (strict)"("Val(Sgnl)"=FALSE) -> ()  [unwired: 2 in, 2 out]
          }
          event "MoveStage": Value Change {
            n142 = event-data() -> ("OldVal"=w309:bool, "NewVal"=w312:bool)  [unwired: 1 in, 4 out]
            n143 = flat-sequence {
              tunnel: w312 -> [w319]
              tunnel: [w319] -> w311
              tunnel: [w316] -> w310
              tunnel: w309 -> [w315]
              tunnel: [w315] -> w308
              tunnel: w311 -> [w322]
              tunnel: w310 -> [w321]
              tunnel: w308 -> [w320]
              frame #0 {
                n144 = call "PasswordPrompt.vi"() -> ("Please enter password below 2"=w318:string)  [unwired: 11 in]
                n145 = Equal?(x=w318, y="l0dat&srv!") -> (x = y?=w316:bool)
              }
              frame #1 {
                n146 = case shown="True" w321 {
                  tunnel: w322 -> [_ w325]
                  tunnel: w320 -> [w323 _]
                  frame False {
                    n147 = call "Display Message to User"("Message"="Wrong Password") -> ()  [unwired: 9 in, 2 out]
                    n148 = property on="MoveStage" class="Bool (strict)"("Value"=w323) -> ()  [unwired: 2 in, 2 out]
                  }
                  frame True {
                    n149 = case shown="True" w325 {
                      frame False {
                        n150 = property on="Position.Ch1::44" class="DigNum (strict)"("Val(Sgnl)"=150.0 ("Value (Signaling)")) -> ()  [unwired: 2 in, 2 out]
                      }
                      frame True {
                        n151 = property on="Position.Ch1::44" class="DigNum (strict)"("Val(Sgnl)"=0.5 ("Value (Signaling)")) -> ()  [unwired: 2 in, 2 out]
                      }
                    }
                    n152 = property on="MoveStage" class="Bool (strict)"("Value"=w325) -> ()  [unwired: 2 in, 2 out]
                  }
                }
              }
            }
            n153 = call <vilib>:"Add State(s) to Queue__jki_lib_state_machine.vi"("State(s) in (\"\")"=w307) -> ("States Out"=w306:string)  [unwired: 14 in]
          }
          event Panel Close? {
            # "Discard the event because we'll close the front panel ourselves in Macro: Exit"
            # "Close Panel button (pressed) Event\n(this executes Macro: Exit to terminate the VI)"
            n154 = event-data() -> ()  [unwired: 1 in, 1 out]
            n155 = event-data("Discard?"=TRUE) -> ()  [unwired: 1 in, 1 out]
            n156 = call <vilib>:"Add State(s) to Queue__jki_lib_state_machine.vi"("State(s) in Front (\"\")"="Macro: Exit", "State(s) in (\"\")"=w333) -> ("States Out"=w332:string)  [unwired: 13 in]
          }
        }
      }
      frame "---------- Core ----------" {
        # "Do not put any code in this frame.\n(it is a separator no-op)"
        n157 = call <vilib>:"Add State(s) to Queue__jki_lib_state_machine.vi"("State(s) in (\"\")"=w337) -> ("States Out"=w336:string)  [unwired: 14 in]
      }
      frame Default {
        w347 = 42 items=["No error", "Argument error", "Memory is full", "Out of zone", "End of file", "File already open", "Generic file I/O error", "File not found", "File permission error", "Disk is full", "Duplicate path", "Too many files open", "System feature not enabled", "Resource file not found", "Cannot add resource", "Resource not found", "Image not found", "Image memory error", "Pen does not exist", "Config type invalid", "Config token not found", "Config parse error", "Config memory error", "Bad external code format", "Bad external code offset", "External code not present", "Null window", "Destroy window error", "Null menu", "Print aborted", "Bad print record", "Print driver error", "Windows error during printing", "Memory error during printing", "Print dialog error", "Generic print error", "Invalid device refnum", "Device not found", "Device parameter error", "Device unit error", "Cannot open device", "Device call aborted", "Generic error", "Cancelled by user", "Object ID too low", "Object ID too high", "Object not in heap", "Unknown heap", "Unknown object (invalid DefProc)", "Unknown object (DefProc not in table)", "Message out of range", "Invalid (null) method", "Unknown message", "Manager call not supported", "Bad address", "Network operation in progress", "Network operation timed out", "Connection is busy", "Network attribute not supported", "Network error", "Address in use", "System out of memory", "Connection aborted", "Connection refused", "Not connected", "Already connected", "Connection closed", "Initialization error (interapplication manager)", "Bad occurrence", "Wait on unbound occurrence handler", "Occurrence queue overflow", "Datalog type conflict", "Unused", "Unrecognized type (interapplication manager)", "Memory corrupt", "Failed to make temporary DLL", "Old CIN version", "Drag socket not found", "Failed to load drop-object", "Failed to register OLE object", "Failed to release OLE object", "Format specifier type mismatch", "Unknown format specifier", "Too few format specifiers", "Too many format specifiers", "Scan failed", "Newer CIN version", "Error converting to variant", "Runtime menu error", "Password tampered", "Variant attribute not found", "Incompatible variant data type", "Event data is not available", "Event Store is not present", "Occurrence is not found", "Event Queue is not created", "Event info is not available", "Refnum passed is NULL", "Error retrieving Class GUID", "Error retrieving CoClass GUID", "Error retrieving TypeLib GUID.", "Bad built application magic bytes.", "Specific driver is different from the specific driver associated with the Logical Name.", "There is no session opened to the class driver.", "Max Error", "MAX - Error with config objects", "MAX - Error loading configuration", "MAX - Group not supported"]
        # "Current State"
        # "Do not delete, rename, or modify this frame.\n(this is used to capture unhandled states and typos)"
        # "Handle mistyped state name (developer tool)"
        n158 = Format Into String(format string="Software Exception: Unhandled State \"%s\"." ("message"), error in=w343, w338) -> (resulting string=w346:string, error out=w345:errorcluster)  [unwired: 1 in]
        n159 = call <vilib>:"Error Cluster From Error Code.vi"("show call chain? (False)"=TRUE, "error in (no error)"=w345, "error message (\"\")"=w346, "error code (0)"=w347) -> ("error out"=w344:errorcluster)  [unwired: 5 in]
        n160 = call <vilib>:"Add State(s) to Queue__jki_lib_state_machine.vi"("State(s) in (\"\")"=w342) -> ("States Out"=w341:string)  [unwired: 14 in]
      }
      frame "Initialize Core Data" {
        # "Do not delete, rename, or modify this frame.\n(this is used to determine panel behavior on exit)"
        # "originally closed?"
        # "exe?"
        # "If panel starts closed or is an EXE, then close it when we exit"
        n161 = property class="VI"() -> ("Front Panel.Open"=w356:bool)  [unwired: 2 in, 2 out]
        n162 = property class="App"() -> ("App.Kind"=w355:T8)  [unwired: 2 in, 2 out]
        n163 = control-ref of="Current VI Reference"() -> (w349:refnum<vi>)
        n164 = Not(x=w356) -> (.not. x?=w353:bool)
        n165 = Equal?(x=w355, y=T8."Run Time System" ("Application:Kind")) -> (x = y?=w352:bool)
        n166 = Or(x=w353, y=w352) -> (x .or. y?=w350:bool)
        n167 = Bundle By Name(cluster=w351, "Core.Current VI Reference"=w349, "Core.Close Panel on Exit?"=w350) -> (w358:T12)
        n168 = call <vilib>:"Add State(s) to Queue__jki_lib_state_machine.vi"("State(s) in (\"\")"=w360) -> ("States Out"=w359:string)  [unwired: 14 in]
      }
      frame "Error Handler" {
        # "Unhandled Error -- Display it"
        # "Handle any errors here.\nYou can also output any states to clean-up after errors occur"
        # "Clear error"
        n169 = call <vilib>:"General Error Handler.vi"("error in (no error)"=w362) -> ()  [unwired: 10 in, 5 out]
        n170 = call <vilib>:"Add State(s) to Queue__jki_lib_state_machine.vi"("State(s) in Front (\"\")"="/* Post Error States", "State(s) in (\"\")"=w366) -> ("States Out"=w365:string)  [unwired: 13 in]
      }
      frame "Exit" {
        # "Do not put any code in this frame.\n(No errors that occur here will be handled.)"
        n171 = call <vilib>:"Add State(s) to Queue__jki_lib_state_machine.vi"("State(s) in (\"\")"=w371) -> ("States Out"=w370:string)  [unwired: 14 in]
      }
      frame "---------- Data ----------" {
        # "Do not put any code in this frame.\n(It is a separator no-op. You can make a copy of this frame to create a new Data frame)"
        n172 = call <vilib>:"Add State(s) to Queue__jki_lib_state_machine.vi"("State(s) in (\"\")"=w375) -> ("States Out"=w374:string)  [unwired: 14 in]
      }
      frame "Data: Initialize" {
        w376 = FALSE  # Fire Continues Allowed
        w378 = u32 0  # Tik1
        w377 = u32 0  # Tik2
        w379 = FALSE  # Jet trigger
        w380 = 0.0  # Discharge timing offset
        w381 = 0.0  # Heater timing offset
        w382 = T13 {"Current VI Reference"=refnum, "Close Panel on Exit?"=FALSE}  # Core
        # "Data names and types of shift register data are defined by this bundle."
        # "Initialize the shift-register data, here.\n(data names are defined by what you wire into the bundle function)"
        n173 = Bundle("Core"=w382, "Heater timing offset"=w381, "Discharge timing offset"=w380, "Jet trigger"=w379, "Tik1"=w378, "Tik2"=w377, "Fire Continues Allowed"=w376) -> (w384:T12)  [unwired: 1 in]
        n174 = call <vilib>:"Add State(s) to Queue__jki_lib_state_machine.vi"("State(s) in (\"\")"=w386) -> ("States Out"=w385:string)  [unwired: 14 in]
      }
      frame "Data: Cleanup" {
        # "Cleanup any data and references, here.\n(this is called automatically, by the Macro: Exit)"
        n175 = Unbundle By Name(w387) -> ("Core.Current VI Reference"=w390:refnum<vi>)
        n176 = Close Reference(reference=w390, error in (no error)=w389) -> (error out=w388:errorcluster)
        n177 = call <vilib>:"Add State(s) to Queue__jki_lib_state_machine.vi"("State(s) in (\"\")"=w392) -> ("States Out"=w391:string)  [unwired: 14 in]
      }
      frame "---------- UI ----------" {
        # "Do not put any code in this frame.\n(It is a separator no-op. You can make a copy of this frame to create a new UI frame)"
        n178 = call <vilib>:"Add State(s) to Queue__jki_lib_state_machine.vi"("State(s) in (\"\")"=w396) -> ("States Out"=w395:string)  [unwired: 14 in]
      }
      frame "UI: Initialize" {
        # "Initialize the User Interface, here.\n(this is called automatically, by the Macro: Init)"
        n179 = call <userlib>:"Fit VI window to Largest Dec__ogtk.vi"() -> ()  [unwired: 6 in, 2 out]
        n180 = call <vilib>:"Add State(s) to Queue__jki_lib_state_machine.vi"("State(s) in (\"\")"=w400) -> ("States Out"=w399:string)  [unwired: 14 in]
      }
      frame "UI: Cursor Set" {
        # "Argument"
        # "Set and Unset Cursor Busy.\n(Usage: \"UI: Cursor Set >> Busy|Idle\")"
        n181 = case shown="\"Idle\", Default" w401 {
          tunnel: w403 -> [w408 w410]
          tunnel: [w407 w409] -> w402
          frame "Idle", Default {
            n182 = call <vilib>:"Unset Busy.vi"("error in (no error)"=w408) -> ("error out"=w407:errorcluster)  [unwired: 10 in]
          }
          frame "Busy" {
            n183 = call <vilib>:"Set Busy.vi"("error in (no error)"=w410) -> ("error out"=w409:errorcluster)  [unwired: 9 in, 1 out]
          }
        }
        n184 = call <vilib>:"Add State(s) to Queue__jki_lib_state_machine.vi"("State(s) in (\"\")"=w406) -> ("States Out"=w405:string)  [unwired: 14 in]
      }
      frame "UI: Front Panel State" {
        # "Argument"
        # "Set Front Panel Open or Closed\n(Usage: \"UI: Front Panel State >> Open|Close\")"
        n185 = Unbundle By Name(w413) -> ("Core.Current VI Reference"=w412:refnum<vi>)
        n186 = case shown="\"Close\"" w411 {
          tunnel: w415 -> [w421 w434]
          tunnel: [w423 w435] -> w414
          tunnel: w412 -> [w422 w432]
          frame "Open", Default {
            n187 = property class="VI"(reference=w422, error in=w421) -> (reference out=w419:refnum<vi>, error out=w420:errorcluster, "Front Panel.Open"=w418:bool)
            n188 = case shown="False" w418 {
              tunnel: [w426 w429] -> w423
              tunnel: w420 -> [w425 w429]
              tunnel: w419 -> [w424 _]
              frame False {
                n189 = invoke class="VI" method="FP.Open"(reference=w424, error in=w425, "Activate"=TRUE, "State"=T9."Standard") -> (error out=w426:errorcluster)  [unwired: 1 in, 4 out]
              }
              frame True {
              }
            }
          }
          frame "Close" {
            n190 = property class="VI"(reference=w432, error in=w434) -> (reference out=w431:refnum<vi>, error out=w433:errorcluster, "Front Panel.Open"=w430:bool)
            n191 = case shown="True" w430 {
              tunnel: [w436 w439] -> w435
              tunnel: w433 -> [w436 w438]
              tunnel: w431 -> [_ w437]
              frame False {
              }
              frame True {
                n192 = invoke class="VI" method="FP.Close"(reference=w437, error in=w438) -> (error out=w439:errorcluster)  [unwired: 1 in, 2 out]
              }
            }
          }
        }
        n193 = call <vilib>:"Add State(s) to Queue__jki_lib_state_machine.vi"("State(s) in (\"\")"=w417) -> ("States Out"=w416:string)  [unwired: 14 in]
      }
      frame "---------- Macro ----------" {
        # "Do not put any code in this frame.\n(It is a separator no-op. You can make a copy of this frame to create a new Macro frame)"
        n194 = call <vilib>:"Add State(s) to Queue__jki_lib_state_machine.vi"("State(s) in (\"\")"=w443) -> ("States Out"=w442:string)  [unwired: 14 in]
      }
      frame "Macro: Initialize" {
        w444 = "Data: Initialize\nInitialize Core Data\nUI: Initialize\nUI: Front Panel State >> Open\nCheck if Fire continues allowed\nInitilize Fire Continues\nInit:MegattenuatorStage"  # Data: Initialize Initialize Core Data UI: Initialize UI: Front Panel State >> Open Check if Fire continues allowed Initilize Fire Continues Init:MegattenuatorStage
        # "Initialization Macro\n(This is called once, when the VI starts)"
        n195 = call <vilib>:"Add State(s) to Queue__jki_lib_state_machine.vi"("State(s) in Front (\"\")"=w444, "State(s) in (\"\")"=w448) -> ("States Out"=w447:string)  [unwired: 13 in]
      }
      frame "Macro: Exit" {
        # "Exit Macro\n(This is called once, when the VI exits)"
        n196 = Unbundle By Name(w458) -> ("Core.Close Panel on Exit?"=w457:bool)
        n197 = Release Queue(queue=w450, force destroy? (F)=TRUE) -> (error out=w449:errorcluster)  [unwired: 1 in, 2 out]
        n198 = call <vilib>:"Clear Errors.vi"("error in (no error)"=w449) -> ()  [unwired: 5 in, 2 out]
        n199 = Select(t="UI: Front Panel State >> Close", s=w457, f="") -> (s? t:f=w454:string)
        n200 = call <vilib>:"Add State(s) to Queue__jki_lib_state_machine.vi"("State(s) in (\"\")"=w454, "State(s) at Back (\"\")"="Data: Cleanup\nExit") -> ("States Out"=w452:string)  [unwired: 13 in]
        n201 = call <vilib>:"Add State(s) to Queue__jki_lib_state_machine.vi"("State(s) in Front (\"\")"=w452, "State(s) in (\"\")"=w461) -> ("States Out"=w460:string)  [unwired: 13 in]
      }
      frame "---------- New Category ----------" {
        # "Template Separator\n(You can make a copy of, or modify, this frame)"
        n202 = call <vilib>:"Add State(s) to Queue__jki_lib_state_machine.vi"("State(s) in (\"\")"=w465) -> ("States Out"=w464:string)  [unwired: 14 in]
      }
      frame "Check Megattenuator Stage Status" {
        n203 = property on="Position.Ch1::44" class="DigNum (strict)"() -> ("Value"=w466:dbl)  [unwired: 2 in, 2 out]
        n204 = case shown="0, 1" w466 {
          tunnel: ["IN" "Unknown/Moving" "OUT"] -> w467
          frame 0, 1 {
            n205 = property on="MoveStage" class="Bool (strict)"("Value"=TRUE) -> ()  [unwired: 2 in, 2 out]
          }
          frame 2, Default {
          }
          frame 149..151 {
            n206 = property on="MoveStage" class="Bool (strict)"("Value"=FALSE) -> ()  [unwired: 2 in, 2 out]
          }
        }
        n207 = property on="CurrentStatus" class="Str"("Value"=w467) -> ()  [unwired: 2 in, 2 out]
        n208 = call <vilib>:"Add State(s) to Queue__jki_lib_state_machine.vi"("State(s) in (\"\")"=w471) -> ("States Out"=w470:string)  [unwired: 14 in]
      }
      frame "Init:MegattenuatorStage" {
        # "Template Separator\n(You can make a copy of, or modify, this frame)"
        n209 = disable-structure shown="Disabled" {
          frame Disabled {
            n210 = flat-sequence {
              frame #0 {
                n211 = call <vilib>:"Set Busy.vi"("disable click? (T)"=TRUE, "cursor ID"=refnum<k1> refnum) -> ()  [unwired: 8 in, 2 out]
              }
              frame #1 {
                n212 = while {
                  tunnel: [w492] -> w484
                  i -> [w487]
                  stop <- w488 stop-if-true
                  n213 = property on="Position.Ch1::44" class="DigNum (strict)"() -> ("Value"=w492:dbl)  [unwired: 2 in, 2 out]
                  n214 = Equal?(x=50, y=w487) -> (x = y?=w485:bool)
                  n215 = Not Equal?(x=w492, y=0.0) -> (x != y?=w489:bool)
                  n216 = Wait (ms)(milliseconds to wait=u32 100) -> ()  [unwired: 1 out]
                  n217 = Or(x=w489, y=w485) -> (x .or. y?=w488:bool)
                }
                n218 = case shown="0, 1" w484 {
                  tunnel: ["IN" "Unknown" "OUT"] -> w483
                  frame 0, 1 {
                    n219 = property on="MoveStage" class="Bool (strict)"("Value"=TRUE) -> ()  [unwired: 2 in, 2 out]
                  }
                  frame 2, Default {
                    n220 = property on="MoveStage" class="Bool (strict)"("DisabledEnum"=T7."Disabled" ("Disabled")) -> ()  [unwired: 2 in, 2 out]
                  }
                  frame 149..151 {
                    n221 = property on="MoveStage" class="Bool (strict)"("Value"=FALSE) -> ()  [unwired: 2 in, 2 out]
                  }
                }
                n222 = property on="CurrentStatus" class="Str"("Value"=w483) -> ()  [unwired: 2 in, 2 out]
              }
              frame #2 {
                n223 = call <vilib>:"Unset Busy.vi"() -> ()  [unwired: 11 in, 1 out]
              }
            }
          }
          frame Enabled {
          }
        }
        n224 = call <vilib>:"Add State(s) to Queue__jki_lib_state_machine.vi"("State(s) in (\"\")"=w480) -> ("States Out"=w479:string)  [unwired: 14 in]
      }
      frame "CheckTimeFire" {
        # "Your code here.\n(You can make a copy of, or modify, this frame)"
        n225 = Unbundle By Name(w505) -> ("Tik1"=w510:u32)
        n226 = Tick Count (ms)() -> (millisecond timer value=w512:u32)
        n227 = Unbundle By Name(w505) -> ("Fire Continues Allowed"=w502:bool)
        n228 = Reciprocal(x="Rate (Hz)") -> (1/x=w501:dbl)
        n229 = Subtract(x=w512, y=w510) -> (x-y=w513:u32)
        n230 = Multiply(x=1000.0, y=w501) -> (x*y=w500:dbl)
        n231 = Greater?(x=w513, y=w500) -> (0:w508:bool)
        n232 = And(x=w508, y="value0::22") -> (x .and. y?=w504:bool)
        n233 = And(x=w502, y=w504) -> (x .and. y?=w503:bool)
        n234 = case shown="True" w503 {
          tunnel: w512 -> [_ w520]
          tunnel: [w518 w520] -> w511
          tunnel: w510 -> [w518 _]
          tunnel: [_ "Action: Fire" ("State(s) in Front (\"\")")] -> w507
          frame False {
          }
          frame True {
          }
        }
        n235 = Bundle By Name(cluster=w505, "Tik1"=w511) -> (w514:T12)
        n236 = call <vilib>:"Add State(s) to Queue__jki_lib_state_machine.vi"("State(s) in Front (\"\")"=w507, "State(s) in (\"\")"=w517) -> ("States Out"=w516:string)  [unwired: 13 in]
        "Fire continues Indicator" <- "value0::22"
      }
      frame "Initilize Fire Continues" {
        # "Your code here.\n(You can make a copy of, or modify, this frame)"
        n237 = Unbundle By Name(w524) -> ("Fire Continues Allowed"=w523:bool)
        n238 = property on="value0::22" class="Bool (strict)"(error in=w526, "Visible"=w523) -> (error out=w525:errorcluster)  [unwired: 1 in, 1 out]
        n239 = Not(x=w523) -> (.not. x?=w521:bool)
        n240 = property on="Fire continues Indicator" class="Bool (strict)"(error in=w525, "Visible"=w521) -> (error out=w522:errorcluster)  [unwired: 1 in, 1 out]
        n241 = call <vilib>:"Add State(s) to Queue__jki_lib_state_machine.vi"("State(s) in (\"\")"=w528) -> ("States Out"=w527:string)  [unwired: 14 in]
      }
      frame "Check if Fire continues allowed" {
        # "Check if it is allowed computer"
        # "Your code here.\n(You can make a copy of, or modify, this frame)"
        n242 = String To IP() -> (0:w536:u32)  [unwired: 1 in]
        n243 = IP To String(1:TRUE ("dot notation? (F)"), 2:w536) -> (0:w537:string)
        n244 = Equal?(x=w537, y="192.168.14.2") -> (x = y?=w531:bool)
        n245 = Not(x=w531) -> (.not. x?=w532:bool)
        n246 = Bundle By Name(cluster=w534, "Fire Continues Allowed"=w531) -> (w533:T12)
        n247 = property on="Allow Fire Continues" class="Bool (strict)"(error in=w530, "Visible"=w532) -> (error out=w529:errorcluster)  [unwired: 1 in, 1 out]
        n248 = call <vilib>:"Add State(s) to Queue__jki_lib_state_machine.vi"("State(s) in (\"\")"=w540) -> ("States Out"=w539:string)  [unwired: 14 in]
      }
      frame "CheckTime2" {
        # "Your code here.\n(You can make a copy of, or modify, this frame)"
        n249 = Unbundle By Name(w549) -> ("Tik2"=w542:u32)
        n250 = Tick Count (ms)() -> (millisecond timer value=w544:u32)
        n251 = Subtract(x=w544, y=w542) -> (x-y=w547:u32)
        n252 = Greater?(x=w547, y=5000) -> (0:w545:bool)
        n253 = case shown="True" w545 {
          tunnel: w544 -> [_ w555]
          tunnel: [w553 w555] -> w543
          tunnel: w542 -> [w553 _]
          tunnel: [_ "Action: update expt vars\nAction: save screenshot"] -> w541
          frame False {
          }
          frame True {
          }
        }
        n254 = Bundle By Name(cluster=w549, "Tik2"=w543) -> (w548:T12)
        n255 = call <vilib>:"Add State(s) to Queue__jki_lib_state_machine.vi"("State(s) in Front (\"\")"=w541, "State(s) in (\"\")"=w552) -> ("States Out"=w551:string)  [unwired: 13 in]
      }
      frame "Action: Fire" {
        n256 = property on="fire::10" class="Str"(error in=w557, "Val(Sgnl)"="fire>>force" ("Value (Signaling)")) -> (error out=w556:errorcluster)  [unwired: 1 in, 1 out]
        n257 = call <vilib>:"Add State(s) to Queue__jki_lib_state_machine.vi"("State(s) in (\"\")"=w561) -> ("States Out"=w560:string)  [unwired: 14 in]
      }
      frame "Action: update expt vars" {
        # "Your code here.\n(You can make a copy of, or modify, this frame)"
        n258 = call <vilib>:"Add State(s) to Queue__jki_lib_state_machine.vi"("State(s) in (\"\")"=w565) -> ("States Out"=w564:string)  [unwired: 14 in]
      }
      frame "Action: SendScanParameters" {
        # "Your code here.\n(You can make a copy of, or modify, this frame)"
        n259 = call "BELLA PW scan mode shot control shutter.vi"("ScanShotControl"="value0::43") -> ("error out"=w569:errorcluster)  [unwired: 10 in]
        n260 = call "Jet in scan on or off.vi"("error in (no error)"=w569, "gas jet on time"="value4::42", "GasJetOn"="value1::43") -> ("error out"=w566:errorcluster)  [unwired: 8 in]
        n261 = flat-sequence {
          tunnel: w566 -> [_]
          frame #0 {
            n262 = One Button Dialog(message="expt editor set up") -> ()  [unwired: 1 in, 1 out]
          }
        }
        n263 = call <vilib>:"Add State(s) to Queue__jki_lib_state_machine.vi"("State(s) in (\"\")"=w574) -> ("States Out"=w573:string)  [unwired: 14 in]
      }
      frame "Action: save screenshot" {
        # "Your code here.\n(You can make a copy of, or modify, this frame)"
        n264 = case shown="True" "Save screenshots" {
          frame False {
          }
          frame True {
            n265 = invoke class="VI" method="FP.Get Image"() -> ("image data"=w583:T10)  [unwired: 6 in, 5 out]
            n266 = call <vilib>:"Write PNG File.vi"("image data"=w583, "path to PNG file"=path "N:/data/ECS dumps/Logmaker Screenshot/frontpanel.png" ("report file path")) -> ("error out"=→"error out":errorcluster)  [unwired: 8 in, 1 out]
          }
        }
        n267 = call <vilib>:"Add State(s) to Queue__jki_lib_state_machine.vi"("State(s) in (\"\")"=w580) -> ("States Out"=w579:string)  [unwired: 14 in]
      }
    }
  }
  n268 = disable-structure shown="Disabled" {
    frame Disabled {
    }
    frame Enabled {
    }
  }
  "CurrentStatus" <- ""
